vi "Fit.vi"(8 "error in (no error)":errorcluster caption="entrée d'erreur (pas d'erreur)", 9 "y":string[][](array[string]), 10 "X":string[][](array[string]), 11 "KernelCenterer.lvclass":refnum<class "KernelCenterer.lvclass">) -> (0 "error out":errorcluster caption="sortie d'erreur", 2 "String Data":string, 3 "KernelCenterer.lvclass":refnum<class "KernelCenterer.lvclass">)   [LabVIEW 2020, in "KernelCenterer.lvclass"]
doc: "Fit KernelCenterer\n\nReturns : \n\n- String : OK"
uses:
  KernelCenterer.lvclass
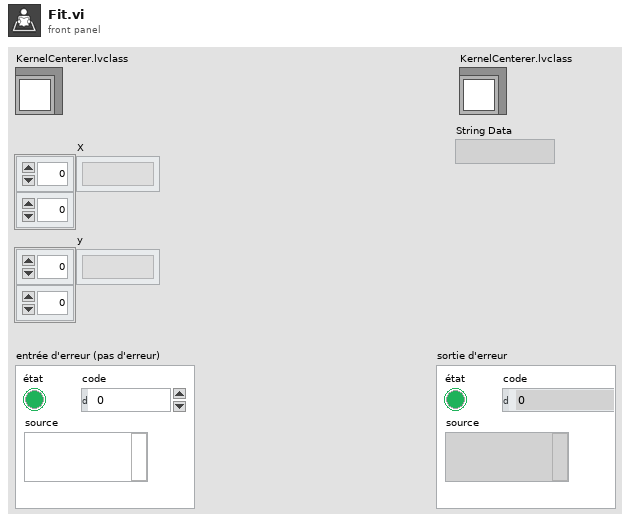
[diagram p1: front panel]
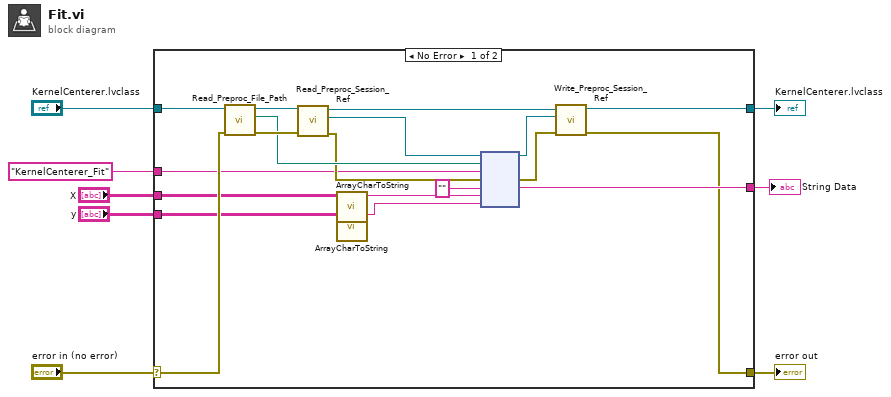
[diagram p0: block diagram]
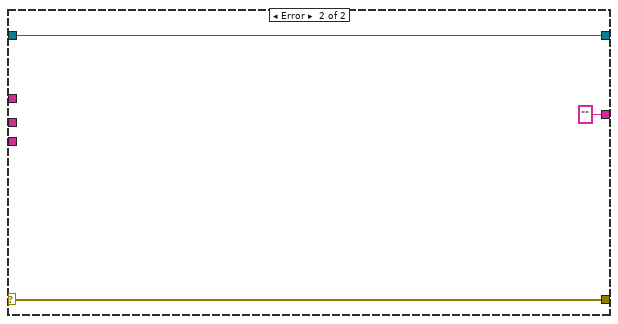
[diagram p2: hidden frame]
diagram:
  n1 = case shown="No Error" "error in (no error)" {
    selector: "error in (no error)" -> [w17 w30]
    tunnel: [w10 w30] -> w7
    tunnel: [w9 w29] -> w5
    tunnel: "KernelCenterer.lvclass" -> [w18 w29]
    tunnel: "KernelCenterer_Fit" ("Fonction") -> [w16 _]
    tunnel: [w15 ""] -> w3
    tunnel: "X" -> [w14 _]
    tunnel: "y" -> [w13 _]
    frame No Error {
      n2 = call-dynamic "Read_Preproc_File_Path.vi"("error in (no error)"=w17, "Python in"=w18) -> ("error out"=w26:errorcluster, "File_Path"=w23:path, "Python out"=w27:refnum<class "KernelCenterer.lvclass">)  [unwired: 7 in]
      n3 = call-dynamic "Read_Preproc_Session_Ref.vi"("error in (no error)"=w26, "Python in"=w27) -> ("error out"=w22:errorcluster, "Session_ref"=w24:refnum<k35>, "Python out"=w25:refnum<class "KernelCenterer.lvclass">)  [unwired: 7 in]
      n4 = call "ArrayCharToString.vi"("TAB"=w14) -> ("Instruction"=w12:string)  [unwired: 10 in]
      n5 = call "ArrayCharToString.vi"("TAB"=w13) -> ("Instruction"=w11:string)  [unwired: 10 in]
      n6 = node(w24, w23, w16, w22, "", w12, w11) -> (w20:refnum<k35>, w21:errorcluster, w15:string)  [unwired: 2 in, 2 out]
      n7 = call-dynamic "Write_Preproc_Session_Ref.vi"("error in (no error)"=w21, "Session_ref"=w20, "Python in"=w25) -> ("error out"=w10:errorcluster, "Python out"=w9:refnum<class "KernelCenterer.lvclass">)  [unwired: 7 in]
    }
    frame Error {
    }
  }
  "error out" <- w7
  "KernelCenterer.lvclass" <- w5
  "String Data" <- w3
